vi "Unit Test - copy state.vi"() -> (3 "Array":T1(array[cluster])=[{"state"="Idle", "error out"={"status"=FALSE, "code"=0, "source"=""}, "Execution:State"=enum."Idle"}, {"state"="CSM Documentation", "error out"={"status"=FALSE, "code"=0, "source"=""}, "Execution:State"=enum."Idle"}, {"state"="VI Reference", "error out"={"status"=FALSE, "code"=0, "source"=""}, "Execution:State"=enum."Idle"}, {"state"="Error Handler", "error out"={"status"=FALSE, "code"=0, "source"=""}, "Execution:State"=enum."Bad"}, {"state"="Critical Error", "error out"={"status"=FALSE, "code"=0, "source"=""}, "Execution:State"=enum."Idle"}, {"state"="Target Timeout Error", "error out"={"status"=FALSE, "code"=0, "source"=""}, "Execution:State"=enum."Idle"}, {"state"="Target Error", "error out"={"status"=FALSE, "code"=0, "source"=""}, "Execution:State"=enum."Idle"}, {"state"="Async Response", "error out"={"status"=FALSE, "code"=0, "source"=""}, "Execution:State"=enum."Idle"}, {"state"="Response", "error out"={"status"=FALSE, "code"=0, "source"=""}, "Execution:State"=enum."Idle"}, {"state"="Async Message Posted", "error out"={"status"=FALSE, "code"=0, "source"=""}, "Execution:State"=enum."Idle"}, {"state"="Initialize Core Data", "error out"={"status"=FALSE, "code"=0, "source"=""}, "Execution:State"=enum."Idle"}, {"state"="Exit", "error out"={"status"=FALSE, "code"=0, "source"=""}, "Execution:State"=enum."Idle"}, {"state"="Data: Initialize", "error out"={"status"=FALSE, "code"=0, "source"=""}, "Execution:State"=enum."Idle"}, {"state"="Data: Update Indicators", "error out"={"status"=FALSE, "code"=0, "source"=""}, "Execution:State"=enum."Idle"}, {"state"="Data: Cleanup", "error out"={"status"=FALSE, "code"=0, "source"=""}, "Execution:State"=enum."Idle"}, {"state"="Macro: Initialize", "error out"={"status"=FALSE, "code"=0, "source"=""}, "Execution:State"=enum."Idle"}, {"state"="Macro: Exit", "error out"={"status"=FALSE, "code"=0, "source"=""}, "Execution:State"=enum."Idle"}, {"state"="API: API1", "error out"={"status"=FALSE, "code"=0, "source"=""}, "Execution:State"=enum."Idle"}, {"state"="API: API2", "error out"={"status"=FALSE, "code"=0, "source"=""}, "Execution:State"=enum."Idle"}, {"state"="Action: action1", "error out"={"status"=FALSE, "code"=0, "source"=""}, "Execution:State"=enum."Idle"}, {"state"="Action: action2", "error out"={"status"=FALSE, "code"=0, "source"=""}, "Execution:State"=enum."Idle"}])   [LabVIEW 2017, in "testcase-csmhelper.lvclass"]
uses:
  testcase-csmhelper.lvclass
  src/user.lib/_NEVSTOP/Communicable State Machine(CSM)/_csmHelper/CSM-Helper.lvclass/CSM-Helper.ctl
  src/user.lib/_NEVSTOP/Communicable State Machine(CSM)/_csmHelper/Properties/Read VI Ref.vi
  src/user.lib/_NEVSTOP/Communicable State Machine(CSM)/_csmHelper/API/Create From VI Reference.vi
  src/user.lib/_NEVSTOP/Communicable State Machine(CSM)/_csmHelper/Properties/Read States.vi
  src/user.lib/_NEVSTOP/Communicable State Machine(CSM)/_csmHelper/API/Start Undo.vi
  src/user.lib/_NEVSTOP/Communicable State Machine(CSM)/_csmHelper/API/Copy State.vi
  src/user.lib/_NEVSTOP/Communicable State Machine(CSM)/_csmHelper/API/Stop Undo.vi
  src/user.lib/_NEVSTOP/Communicable State Machine(CSM)/_csmHelper/API/Undo.vi
  src/user.lib/_NEVSTOP/Communicable State Machine(CSM)/_csmHelper/API/Destroy.vi
  src/user.lib/_NEVSTOP/Communicable State Machine(CSM)/_csmHelper/CSM-Helper.lvclass
  src/user.lib/_NEVSTOP/Communicable State Machine(CSM)/_csmHelper/API/Open Block Diagram.vi
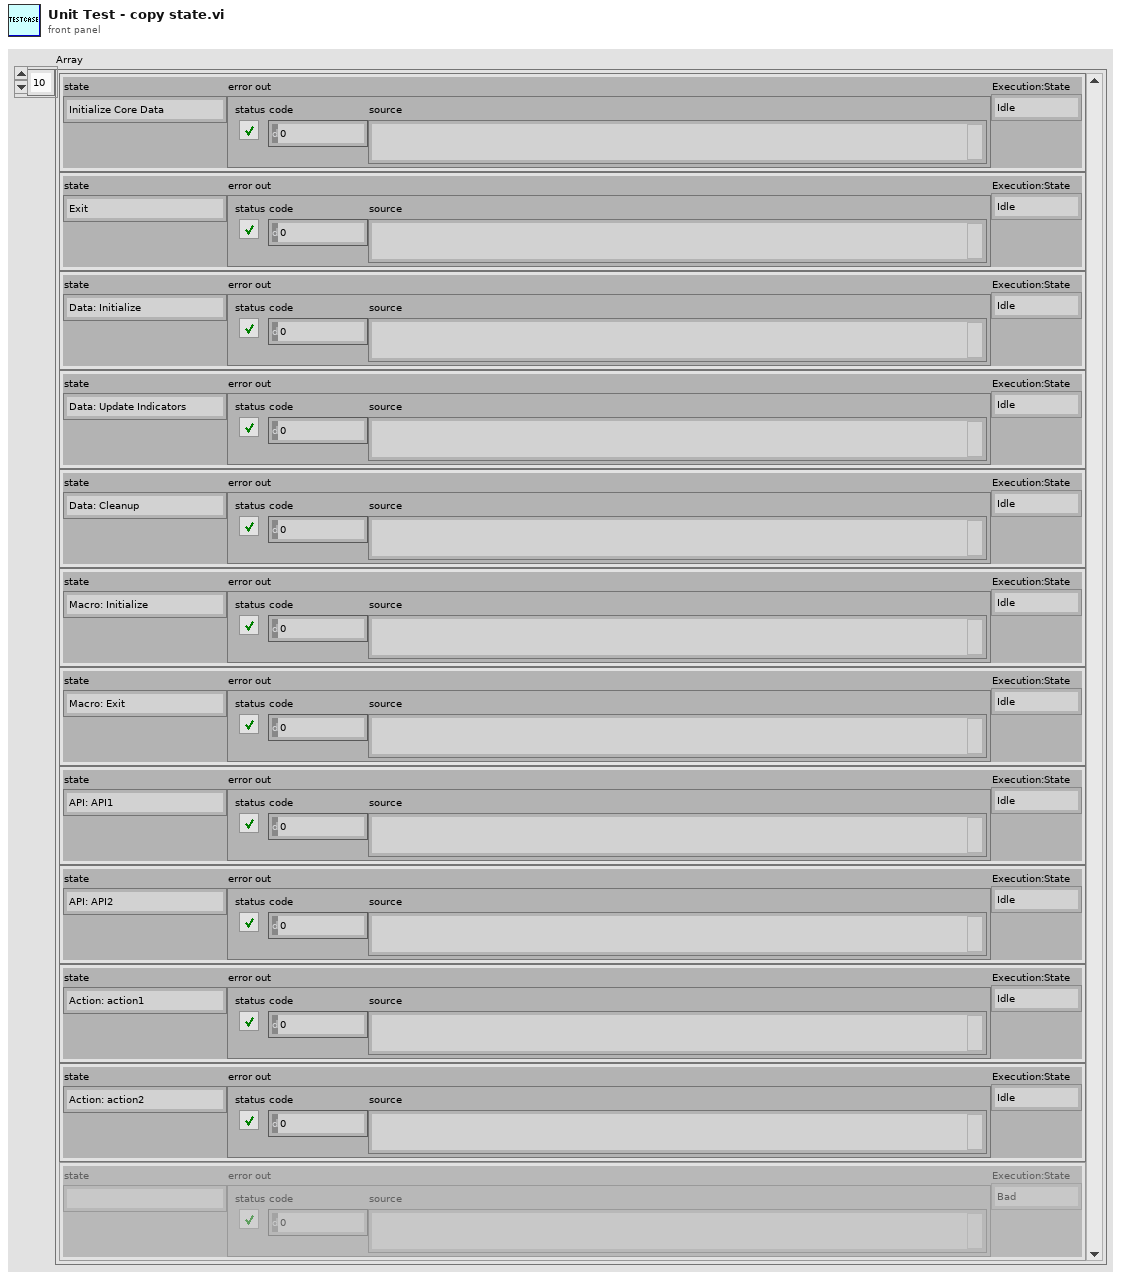
[diagram p1: front panel]
types:
  T1 = cluster{"state":string, "error out":errorcluster, "Execution:State":enum32{"Bad", "Idle", "Run top level", "Running"}}[]
  T2 = enum32{"Bad", "Idle", "Run top level", "Running"}
  T3 = cluster{string, "error out":errorcluster, "Exec.State":enum32{"Bad", "Idle", "Run top level", "Running"}}
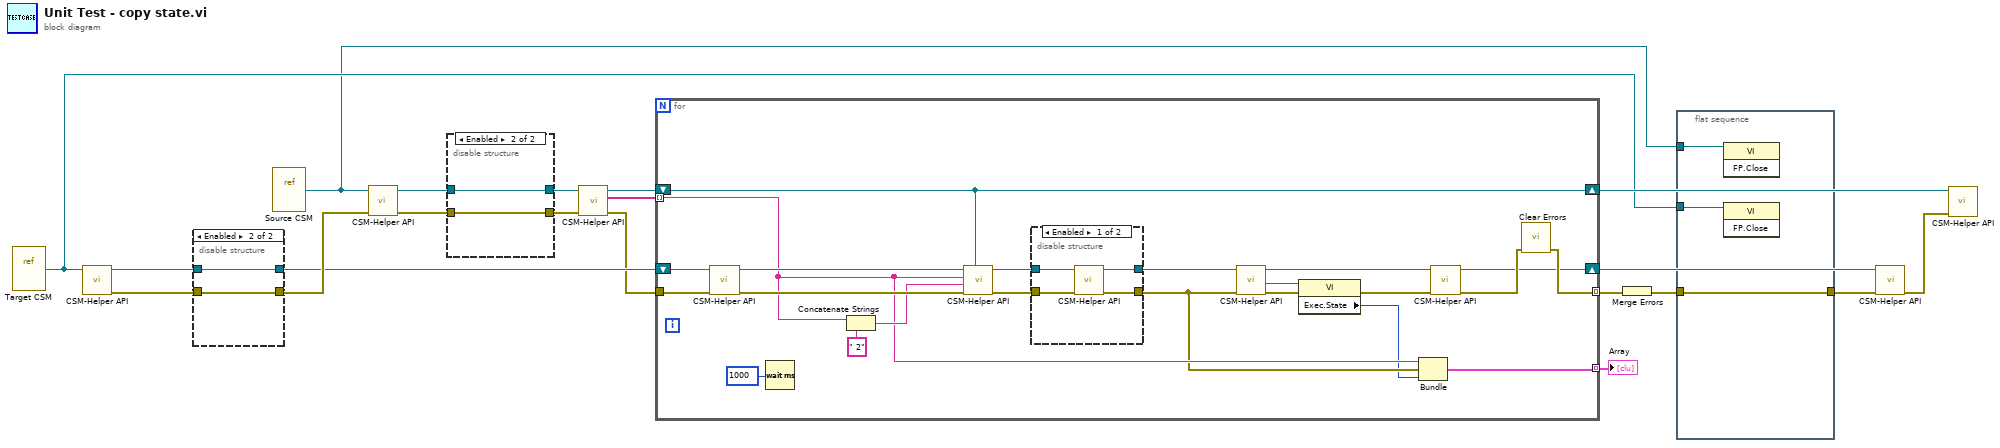
[diagram p0: block diagram]
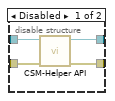
[diagram p2: hidden frame]
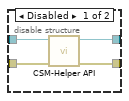
[diagram p3: hidden frame]
diagram:
  n1 = vi-ref "Target CSM.vi"() -> (w2:refnum<vi>)
  n2 = call-poly "CSM-Helper API.vi"("VI"=w2) -> ("error out"=w18:errorcluster, "CSM-Helper.lvclass"=w17:refnum<class "CSM-Helper.lvclass">)  [unwired: 9 in]
  n3 = disable-structure shown="Enabled" {
    disable-tunnel: w18 -> [w24 w26]
    disable-tunnel: w17 -> [w23 w25]
    disable-tunnel: [w22 w26] -> w12
    disable-tunnel: [w21 w25] -> w11
    frame Disabled {
      n4 = call-poly "CSM-Helper API.vi"("error in (no error)"=w24, "CSM-Helper in"=w23) -> ("error out"=w22:errorcluster, "CSM-Helper out"=w21:refnum<class "CSM-Helper.lvclass">)  [unwired: 8 in]
    }
    frame Enabled {
    }
  }
  n5 = vi-ref "Source CSM.vi"() -> (w1:refnum<vi>)
  n6 = call-poly "CSM-Helper API.vi"("error in (no error)"=w12, "VI"=w1) -> ("error out"=w15:errorcluster, "CSM-Helper.lvclass"=w16:refnum<class "CSM-Helper.lvclass">)  [unwired: 8 in]
  n7 = disable-structure shown="Enabled" {
    disable-tunnel: w16 -> [w30 w32]
    disable-tunnel: w15 -> [w29 w31]
    disable-tunnel: [w28 w31] -> w14
    disable-tunnel: [w27 w32] -> w13
    frame Disabled {
      n8 = call-poly "CSM-Helper API.vi"("error in (no error)"=w29, "CSM-Helper in"=w30) -> ("error out"=w28:errorcluster, "CSM-Helper out"=w27:refnum<class "CSM-Helper.lvclass">)  [unwired: 8 in]
    }
    frame Enabled {
    }
  }
  n9 = call-poly "CSM-Helper API.vi"("error in (no error)"=w14, "CSM-Helper in"=w13) -> ("error out"=w10:errorcluster, "Value"=w6:string[], "CSM-Helper out"=w9:refnum<class "CSM-Helper.lvclass">)  [unwired: 7 in]
  n10 = for {
    shift-right: [w40] -> w20
    shift-left: w11 -> [w53]
    shift-right: [w48] -> w7
    shift-left: w9 -> [w48]
    tunnel: w6 -> [w44] mode=indexing
    tunnel: w10 -> [w52]
    tunnel: [w45] -> w19 mode=indexing
    tunnel: [w43] -> w5 mode=indexing
    n11 = call-poly "CSM-Helper API.vi"("error in (no error)"=w52, "CSM-Helper in"=w53) -> ("error out"=w51:errorcluster, "CSM-Helper out"=w50:refnum<class "CSM-Helper.lvclass">)  [unwired: 8 in]
    n12 = Wait (ms)(milliseconds to wait=u32 1000) -> ()  [unwired: 1 out]
    n13 = Concatenate Strings(w44, " 2" ("string")) -> (w47:string)
    n14 = call-poly "CSM-Helper API.vi"("SourceCSM"=w48, "error in (no error)"=w51, "New(Empty to Use same Name)"=w47, "Case"=w44, "CSM-Helper.lvclass"=w50) -> ("error out"=w49:errorcluster, "CSM-Helper out 2"=w54:refnum<class "CSM-Helper.lvclass">)  [unwired: 5 in]
    n15 = disable-structure shown="Enabled" {
      disable-tunnel: [w58 w60] -> w38
      disable-tunnel: w49 -> [w57 w59]
      disable-tunnel: [w56 w59] -> w39
      disable-tunnel: w54 -> [w55 w60]
      frame Enabled {
        n16 = call-poly "CSM-Helper API.vi"("error in (no error)"=w57, "CSM-Helper in"=w55) -> ("error out"=w56:errorcluster, "CSM-Helper out"=w58:refnum<class "CSM-Helper.lvclass">)  [unwired: 8 in]
      }
      frame Disabled {
      }
    }
    n17 = call-poly "CSM-Helper API.vi"("error in (no error)"=w39, "CSM-Helper in"=w38) -> ("error out"=w36:errorcluster, "VI"=w34:refnum<vi>, "CSM-Helper out"=w37:refnum<class "CSM-Helper.lvclass">)  [unwired: 7 in]
    n18 = property class="VI"(reference=w34, error in=w36) -> (error out=w35:errorcluster, "Exec.State"=w33:T2)  [unwired: 1 out]
    n19 = Bundle(w44, "error out"=w39, "Exec.State"=w33) -> (w43:T3)  [unwired: 1 in]
    n20 = call-poly "CSM-Helper API.vi"("error in (no error)"=w35, "CSM-Helper in"=w37) -> ("error out"=w41:errorcluster, "CSM-Helper out"=w40:refnum<class "CSM-Helper.lvclass">)  [unwired: 8 in]
    n21 = call <vilib>:"Clear Errors.vi"("error in (no error)"=w41) -> ("error out"=w45:errorcluster)  [unwired: 5 in, 1 out]
  }
  "Array" <- w5
  n22 = Merge Errors(w19) -> (w3:errorcluster)
  n23 = flat-sequence {
    tunnel: [w63] -> w4
    tunnel: w3 -> [w63]
    tunnel: w2 -> [w62]
    tunnel: w1 -> [w61]
    frame #0 {
      n24 = invoke class="VI" method="FP.Close"(reference=w61) -> ()  [unwired: 2 in, 3 out]
      n25 = invoke class="VI" method="FP.Close"(reference=w62) -> ()  [unwired: 2 in, 3 out]
    }
  }
  n26 = call-poly "CSM-Helper API.vi"("error in (no error)"=w4, "CSM-Helper in"=w20) -> ("error out"=w8:errorcluster)  [unwired: 8 in, 1 out]
  n27 = call-poly "CSM-Helper API.vi"("error in (no error)"=w8, "CSM-Helper in"=w7) -> ()  [unwired: 8 in, 2 out]
